vi "MainAmmeterComm.vi"() -> ()   [LabVIEW 2010]
uses:
  BaudRate.ctl
  VarableID.ctl
panel:
  in  "视在功率":bool
  in  "功率因数":bool
  in  "电压":bool
  in  "电流":bool
  in  "退出系统":bool
  in  "软件使用说明":bool
  in  "启动采集":bool=TRUE
  in  "baud rate":T1=2400 caption="波特率" items=["1200"=1200, "2400"=2400, "4800"=4800, "9600"=9600, "19200"=19200, "38400"=38400, "115200"=115200, ""=0]
  out "测量变量显示":dbl[][](graph)
  # "智能电表信息采集系统"
  # "信号采集选项"
  # "端口参数设置"
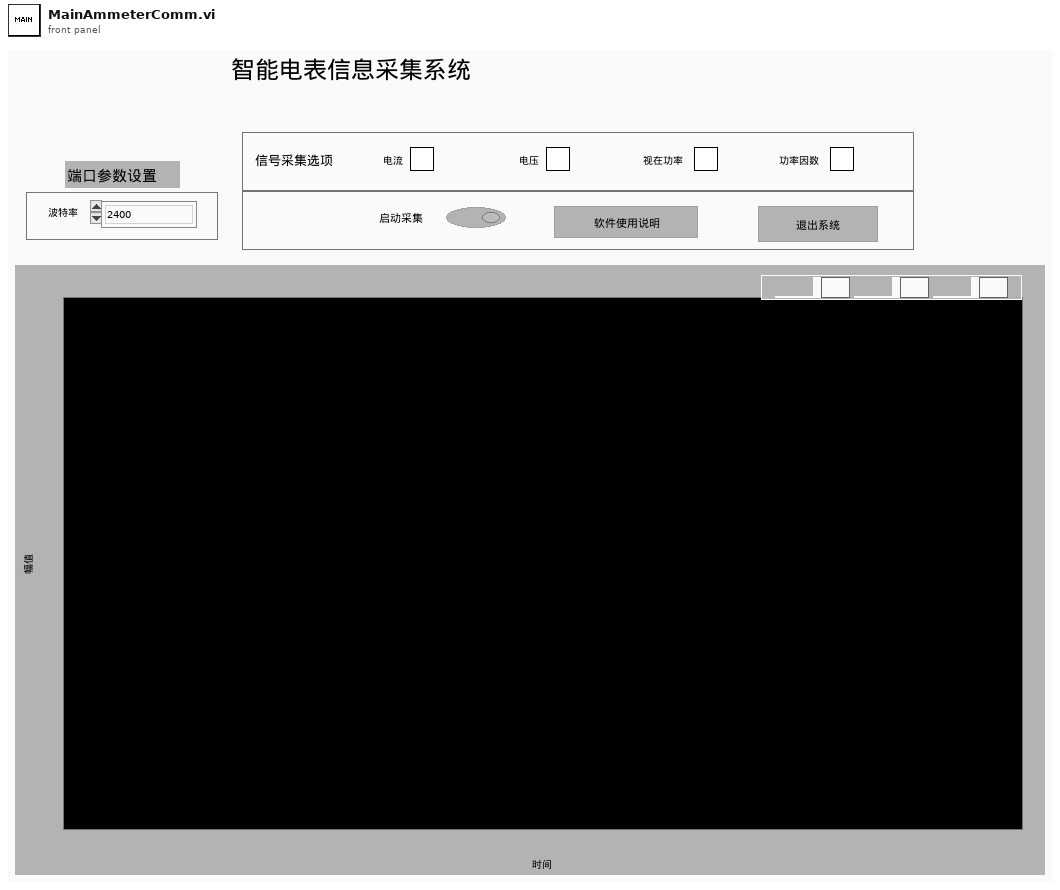
[diagram p1: front panel]
types:
  T1 = typedef "BaudRate.ctl" = u64
  T2 = typedef "OutputDataFormat.ctl" = cluster{"property":string, "dataIdentity":string, "value":string, "address":string}
  T3 = typedef "VarableID.ctl" = enum16{"current", "voltage", "power", "PF"}
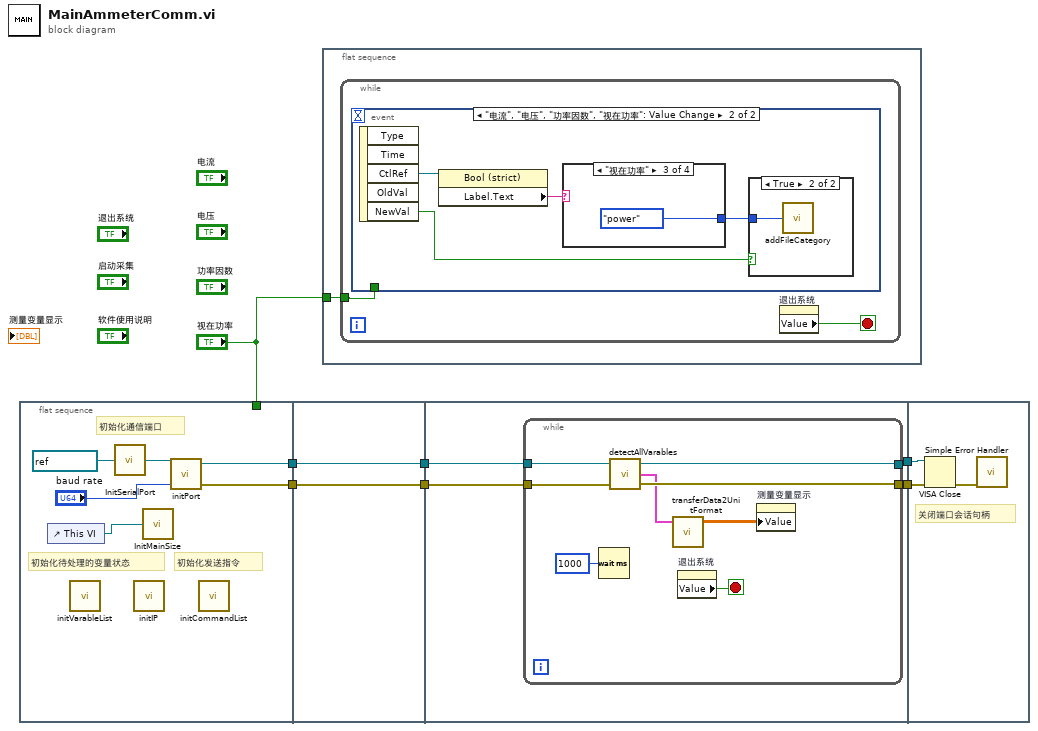
[diagram p0: block diagram]
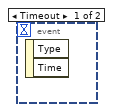
[diagram p2: hidden frame]
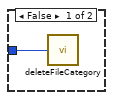
[diagram p3: hidden frame]
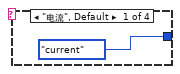
[diagram p4: hidden frame]
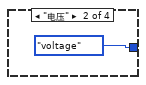
[diagram p5: hidden frame]
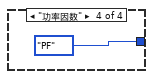
[diagram p6: hidden frame]
diagram:
  n1 = flat-sequence {
    tunnel: [w11] -> w3
    tunnel: "视在功率" -> [_]
    tunnel: [w12] -> w2
    tunnel: [w15] -> w4
    tunnel: w3 -> [w14]
    tunnel: w2 -> [w15]
    tunnel: [w14] -> w1
    tunnel: w4 -> [w19]
    tunnel: [w18] -> w7
    tunnel: [w17] -> w6
    tunnel: w1 -> [w16]
    tunnel: w7 -> [w29]
    tunnel: w6 -> [w28]
    frame #0 {
      # "初始化发送指令"
      # "初始化通信端口"
      # "初始化待处理的变量状态"
      n2 = control-ref of="This VI"() -> (w8:refnum<vi>)
      n3 = call "initVarableList.vi"() -> ()  [unwired: 12 in]
      n4 = call "InitSerialPort.vi"("default resource name"=refnum<visa-resource-name> "COM7" ("Port")) -> ("VISA resource name out"=w9:refnum<visa-resource-name>)
      n5 = call "initIP.vi"() -> ()  [unwired: 12 in]
      n6 = call "InitMainSize.vi"("VI Refnum In"=w8) -> ()  [unwired: 1 out]
      n7 = call "initPort.vi"("baud rate"="baud rate", "VISA resource name"=w9) -> ("error out"=w12:errorcluster, "reference out"=w11:refnum<visa-resource-name>)  [unwired: 2 in]
      n8 = call "initCommandList.vi"() -> ()  [unwired: 12 in]
    }
    frame #1 {
    }
    frame #2 {
      n9 = while {
        tunnel: w19 -> [w23]
        tunnel: [w24] -> w18
        tunnel: [w26] -> w17
        tunnel: w16 -> [w25]
        stop <- w27 stop-if-true
        n10 = Wait (ms)(milliseconds to wait=u32 1000) -> ()  [unwired: 1 out]
        n11 = call "detectAllVarables.vi"("error in (no error)"=w23, "VISA resource name"=w25) -> ("error out"=w26:errorcluster, "Data"=w22:T2[], "VISA resource name 2"=w24:refnum<visa-resource-name>)  [unwired: 1 in]
        n12 = call "transferData2UnitFormat.vi"("Data"=w22) -> ("display"=w21:dbl[][])  [unwired: 4 in]
        n13 = property on="退出系统" class="Bool (strict)"() -> ("Value"=w27:bool)  [unwired: 2 in, 2 out]
        n14 = property on="测量变量显示" class="WFChart (strict)"("Value"=w21) -> ()  [unwired: 2 in, 2 out]
      }
    }
    frame #3 {
      # "关闭端口会话句柄"
      n15 = VISA Close(VISA resource name=w29, error in (no error)=w28) -> (error out=w30:errorcluster)
      n16 = call <vilib>:"Simple Error Handler.vi"("error in (no error)"=w30) -> ()  [unwired: 1 in, 8 out]
    }
  }
  n17 = flat-sequence {
    tunnel: "视在功率" -> [w31]
    frame #0 {
      n18 = while {
        tunnel: w31 -> [w33]
        stop <- w32 stop-if-true
        n19 = event shown="[1] \"电流\", \"电压\", \"功率因数\", \"视在功率\": Value Change" {
          selector: _ -> [_ _]
          dyn-events: _ -> [_ _]
          timeout: _ -> [_ _]
          tunnel: w33 -> [_ _]
          event Timeout {
            n20 = event-data() -> ()  [unwired: 1 in, 2 out]
          }
          event "电流", "电压", "功率因数", "视在功率": Value Change {
            n21 = event-data() -> ("CtlRef"=w34:refnum<vi>, "NewVal"=w35:bool)  [unwired: 1 in, 3 out]
            n22 = property class="Bool (strict)"(reference=w34) -> ("Label.Text"=w37:string)  [unwired: 1 in, 2 out]
            n23 = case shown="\"视在功率\"" w37 {
              tunnel: [VarableID."current" ("VarableID") VarableID."voltage" ("VarableID") VarableID."power" ("VarableID") VarableID."PF" ("VarableID")] -> w36
              frame "电流", Default {
              }
              frame "电压" {
              }
              frame "视在功率" {
              }
              frame "功率因数" {
              }
            }
            n24 = case shown="True" w35 {
              tunnel: w36 -> [w38 w39]
              frame False {
                n25 = call "deleteFileCategory.vi"("VarableID"=w38) -> ()  [unwired: 1 in]
              }
              frame True {
                n26 = call "addFileCategory.vi"("VarableID"=w39) -> ()  [unwired: 1 in]
              }
            }
          }
        }
        n27 = property on="退出系统" class="Bool (strict)"() -> ("Value"=w32:bool)  [unwired: 2 in, 2 out]
      }
    }
  }
